vi "Joystick Sensitivity.vi"(7 "max power (1)":dbl=1.0, 8 "joystick deadband":dbl=0.15, 9 "motor deadband (0.15)":dbl=0.15, 10 "sensitivity (0.5)":dbl=0.5, 11 "x":dbl) -> (2 "Outside Deadband?":bool, 3 "y":dbl)   [LabVIEW 2016]
panel:
  # "Joystick Input"
  # "Joystick output"
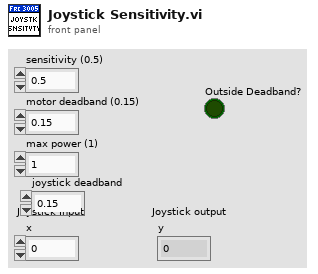
[diagram p1: front panel]
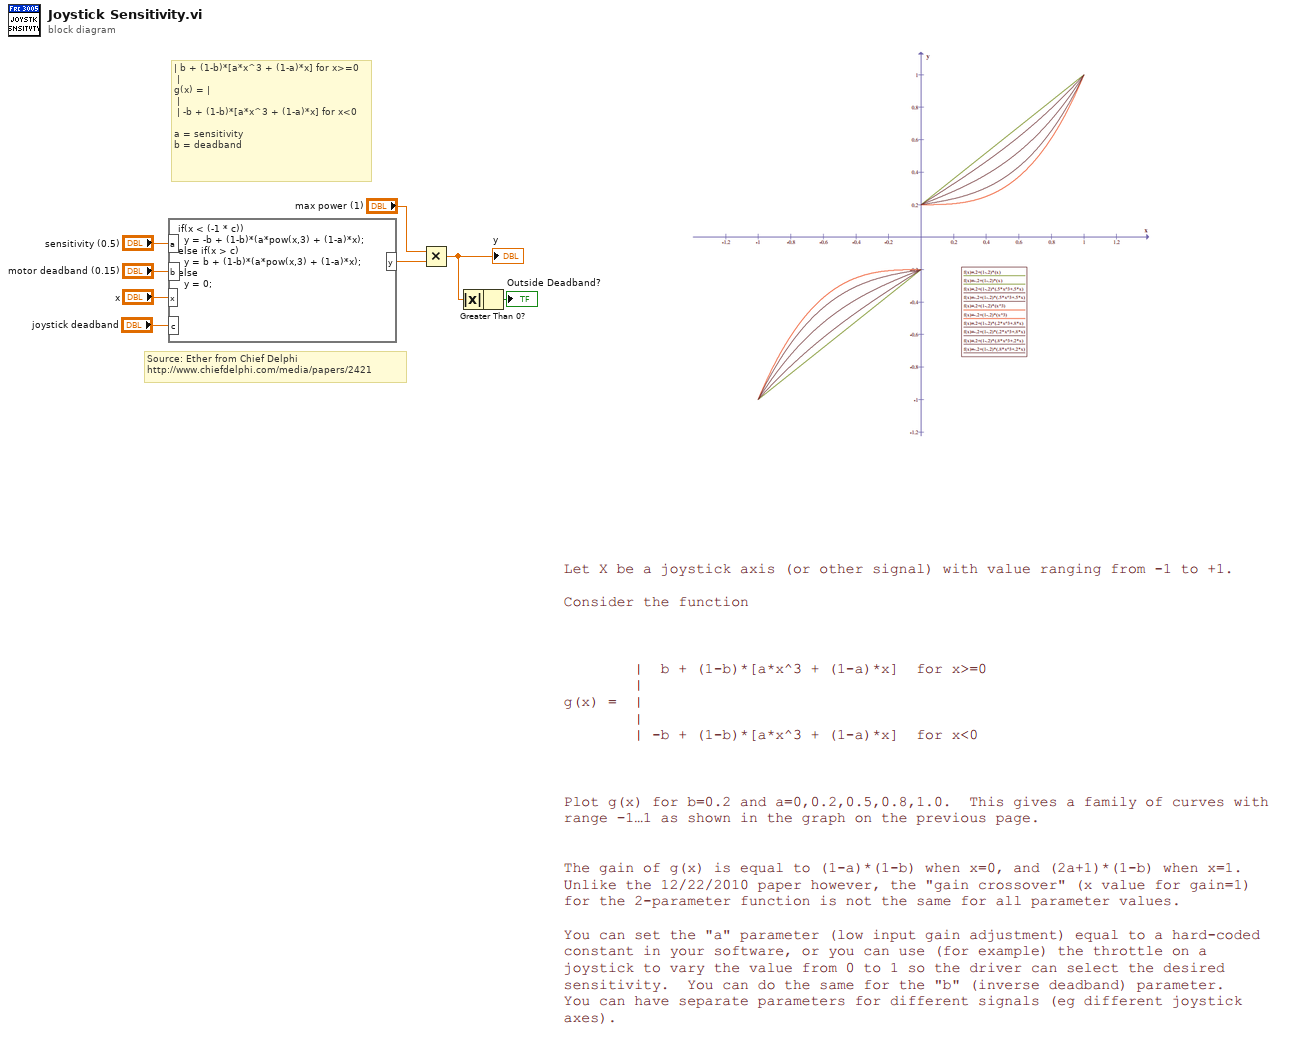
[diagram p0: block diagram]
diagram:
  # "Source: Ether from Chief Delphi\nhttp://www.chiefdelphi.com/media/papers/2421"
  # "| b + (1-b)*[a*x^3 + (1-a)*x] for x>=0\n |\ng(x) = |\n |\n | -b + (1-b)*[a*x^3 + (1-a)*x] for x<0 \n\na = sensitivity\nb = deadband"
  n1 = formula code="if(x < (-1 * c))\n  y = -b + (1-b)*(a*pow(x,3) + (1-a)*x);\nelse if(x > c)\n  y = b + (1-b)*(a*pow(x,3) + (1-a)*x);\nelse\n  y = 0;"("a"="sensitivity (0.5)", "x"="x", "b"="motor deadband (0.15)", "c"="joystick deadband") -> ("y"=w8:dbl)
  n2 = Multiply(x="max power (1)", y=w8) -> (x*y=w6:dbl)
  "y" <- w6
  n3 = Absolute Value(x=w6) -> (abs(x)=w1:dbl)
  n4 = Greater Than 0?(x=w1) -> (x > 0?=→"Outside Deadband?":bool)
